vi "Initialize.vi"(8 "error in (no error)":errorcluster, 11 "TCP in":refnum<class "TCP.lvclass">) -> (0 "error out":errorcluster, 3 "TCP out":refnum<class "TCP.lvclass">)   [LabVIEW 2021, in "TCP.lvclass"]
uses:
  TCP.lvclass
  D:/my_projects/projects/Algorithms/Labview/21/Master CR/Master CR.lvclass
  Param/TCP Param/TCP Param.lvclass
  ctl/MB timeouts.ctl
  Modbus_v121c/Transmission Data Unit/IP/IP Data Unit.lvclass
  D:/my_projects/projects/Algorithms/Labview/21/Modbus_v121c/Transmission Data Unit/Transmission Data Unit.lvclass
  Modbus_v121c/Network Protocol/Network Master/TCP/TCP Master.lvclass
  D:/my_projects/projects/Algorithms/Labview/21/Modbus_v121c/Network Protocol/Network Master/Network Master.lvclass
  D:/my_projects/projects/Algorithms/Labview/21/Modbus_v121c/Network Protocol/Network Protocol.lvclass
  Modbus_v121c/Master Function Definition/Master Function Definition.lvclass
  Master CR.lvclass/Master CR.ctl
  Param/TCP Param/TCP Param.lvclass/TCP Param.ctl
  Modbus_v121c/Transmission Data Unit/IP/IP Data Unit.lvclass/IP Data Unit.ctl
  Modbus_v121c/Transmission Data Unit/Transmission Data Unit.lvclass/Transmission Data Unit.ctl
  Modbus_v121c/Network Protocol/Network Master/Network Master.lvclass/Network Master.ctl
  Modbus_v121c/Transmission Data Unit/IP/Write address.vi
  Modbus_v121c/Transmission Data Unit/IP/Write port.vi
  Modbus_v121c/Transmission Data Unit/IP/Write connect timeout.vi
  Master CR.lvclass
  TCP.lvclass/TCP.ctl
  Modbus_v121c/Transmission Data Unit/Transmission Data Unit.lvclass
  Modbus_v121c/Network Protocol/Network Master/Network Master.lvclass
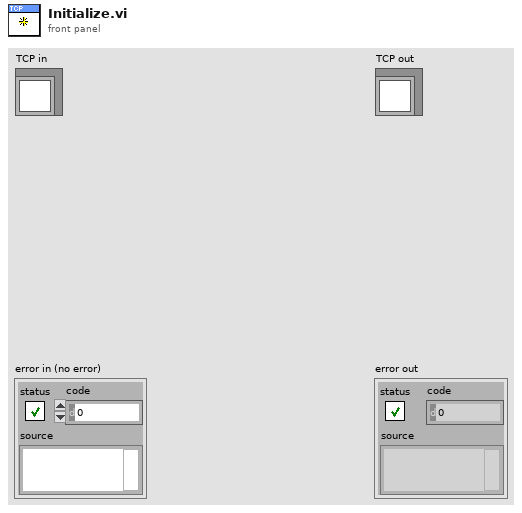
[diagram p1: front panel]
types:
  T1 = typedef "Master CR.lvclass/MB timeouts.ctl" = cluster{"reconn_timeout":i32, "N attempt max":i32, "t_reset_TTL":i32, "period":i32}
  T2 = typedef "Param.lvlib/TCP Param.lvclass/timeouts.ctl" = cluster{"conn_timeout":i32, "reconn_timeout":i32, "N attempt max":i32, "t_reset_TTL":i32, "write_timeout":i32, "read_timeout":i32, "period":i32}
  T3 = cluster{"Remote IP Address":string, "Remote Port":u16}
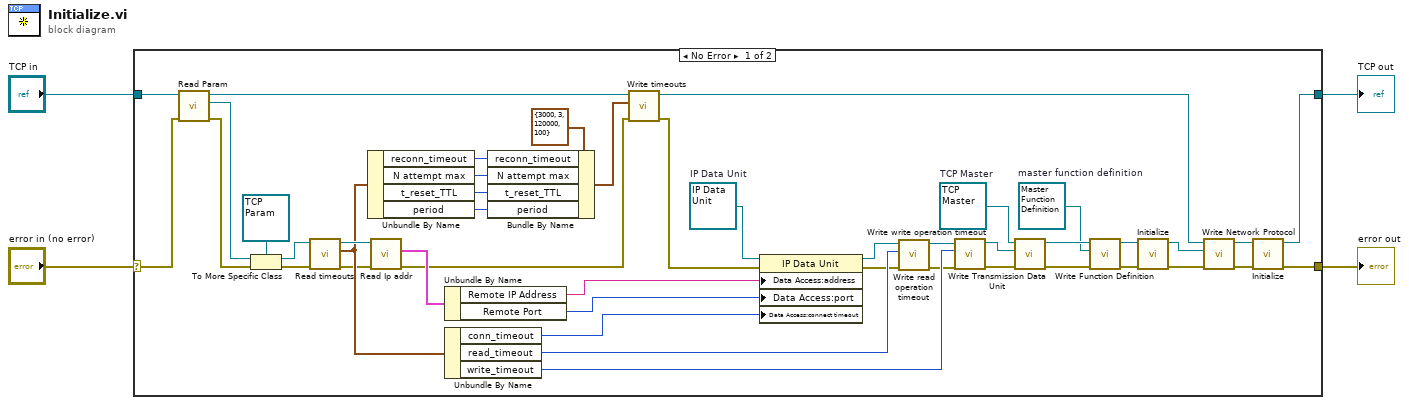
[diagram p0: block diagram]
diagram:
  n1 = case shown="No Error" "error in (no error)" {
    selector: "error in (no error)" -> [w39 w50]
    tunnel: [w29 w50] -> w3
    tunnel: [w30 w51] -> w1
    tunnel: "TCP in" -> [w36 w51]
    frame No Error {
      w5 = refnum<class "Master Function Definition.lvclass"> refnum  # master function definition
      w22 = refnum<class "TCP Master.lvclass"> refnum  # TCP Master
      w16 = refnum<class "IP Data Unit.lvclass"> refnum  # IP Data Unit
      n2 = call "Read Param.vi"("error in (no error)"=w39, "MB_TCP in"=w36) -> ("error out"=w38:errorcluster, "Param"=w35:refnum<class "Param.lvclass">, "MB_TCP out"=w34:refnum<class "TCP.lvclass">)  [unwired: 7 in]
      n3 = To More Specific Class(target class=refnum<class "TCP Param.lvclass"> refnum ("Param.lvlib:TCP Param.lvclass"), reference=w35, error in=w38) -> (specific class reference=w37:refnum<class "TCP Param.lvclass">, error out=w48:errorcluster)
      n4 = call "Read timeouts.vi"("error in (no error)"=w48, "MBParam in"=w37) -> ("error out"=w32:errorcluster, "timeouts"=w33:T2, "MBParam out"=w41:refnum<class "TCP Param.lvclass">)  [unwired: 7 in]
      n5 = Unbundle By Name(w33) -> ("reconn_timeout"=w46:i32, "N attempt max"=w43:i32, "t_reset_TTL"=w44:i32, "period"=w45:i32)
      n6 = call "Read Ip addr.vi"("error in (no error)"=w32, "MBParam in"=w41) -> ("error out"=w31:errorcluster, "IP address"=w40:T3)  [unwired: 7 in, 1 out]
      n7 = Unbundle By Name(w40) -> ("Remote IP Address"=w14:string, "Remote Port"=w13:u16)
      n8 = Unbundle By Name(w33) -> ("conn_timeout"=w12:i32, "read_timeout"=w28:i32, "write_timeout"=w27:i32)
      n9 = Bundle By Name(cluster=T1 {"reconn_timeout"=3000, "N attempt max"=3, "t_reset_TTL"=120000, "period"=100} ("MB timeouts"), "reconn_timeout"=w46, "N attempt max"=w43, "t_reset_TTL"=w44, "period"=w45) -> (w42:T1)
      n10 = call "Write timeouts.vi"("error in (no error)"=w31, "MB timeouts"=w42, "Master CR in"=w34) -> ("error out"=w15:errorcluster, "Master CR out"=w19:refnum<class "TCP.lvclass">)  [unwired: 7 in]
      n11 = property class="IP Data Unit"(reference=w16, error in=w15, "Data Access:address"=w14, "Data Access:port"=w13, "Data Access:connect timeout"=w12) -> (reference out=w10:refnum<class "IP Data Unit.lvclass">, error out=w11:errorcluster)
      n12 = call "Write read operation timeout.vi"("error in (no error)"=w11, "read operation timeout"=w28, "transmission data unit in"=w10) -> ("error out"=w23:errorcluster, "transmission data unit out"=w26:refnum<class "IP Data Unit.lvclass">)  [unwired: 7 in]
      n13 = call "Write write operation timeout.vi"("error in (no error)"=w23, "write operation timeout"=w27, "transmission data unit in"=w26) -> ("error out"=w25:errorcluster, "transmission data unit out"=w24:refnum<class "IP Data Unit.lvclass">)  [unwired: 7 in]
      n14 = call "Write Transmission Data Unit.vi"("error in (no error)"=w25, "Transmission Data Unit"=w24, "Network Master in"=w22) -> ("error out"=w9:errorcluster, "Network Master out"=w6:refnum<class "TCP Master.lvclass">)  [unwired: 7 in]
      n15 = call "Write Function Definition.vi"("error in"=w9, "master function definition"=w5, "Modbus master in"=w6) -> ("error out"=w8:errorcluster, "Modbus master out"=w7:refnum<class "TCP Master.lvclass">)  [unwired: 7 in]
      n16 = call-dynamic "Initialize.vi"("error in"=w8, "TCP master in"=w7) -> ("error out"=w21:errorcluster, "TCP master out"=w20:refnum<class "TCP Master.lvclass">)  [unwired: 8 in]
      n17 = call "Write Network Protocol.vi"("error in (no error)"=w21, "Network Protocol"=w20, "Master CR in"=w19) -> ("error out"=w18:errorcluster, "Master CR out"=w17:refnum<class "TCP.lvclass">)  [unwired: 7 in]
      n18 = call-parent "Initialize.vi"("error in (no error)"=w18, "MB in"=w17) -> ("error out"=w29:errorcluster, "MB out"=w30:refnum<class "TCP.lvclass">)  [unwired: 8 in]
    }
    frame Error {
    }
  }
  "error out" <- w3
  "TCP out" <- w1
